vi "analog write with coercion.vi"(6 "write?":bool=TRUE, 8 "error in (no error)":errorcluster, 10 "data":dbl format="%0.2f", 11 "task/channels in":refnum<k21>) -> (0 "error out":errorcluster, 3 "task out":refnum<k21>)   [LabVIEW 2013]
uses:
  <vilib>/DAQmx/write.llb/DAQmx Write (Analog DBL 1Chan 1Samp).vi
  <vilib>/DAQmx/miscellaneous.llb/DAQmx Fill In Error Info.vi
  <resource>/objmgr/daqmx.rc
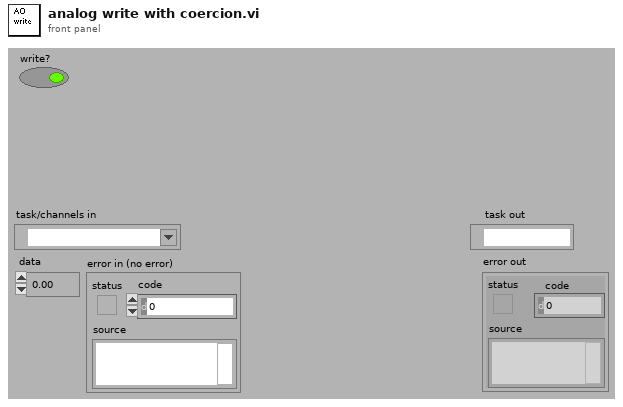
[diagram p1: front panel]
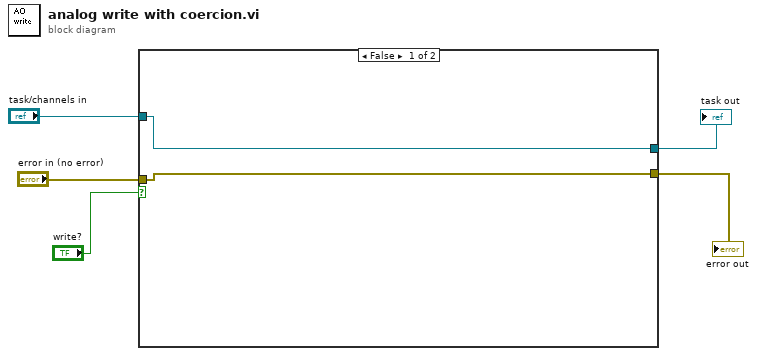
[diagram p0: block diagram]
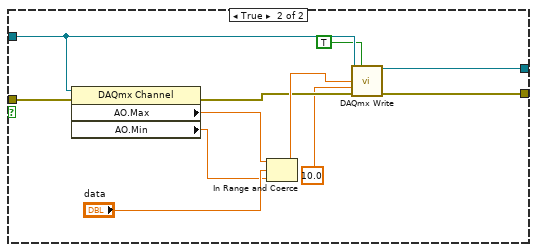
[diagram p2: hidden frame]
diagram:
  n1 = case shown="False" "write?" {
    tunnel: "task/channels in" -> [w7 w18]
    tunnel: [w7 w11] -> w4
    tunnel: [w6 w10] -> w3
    tunnel: "error in (no error)" -> [w6 w8]
    frame False {
    }
    frame True {
      n2 = property class="DAQmx Channel"(reference=w18, error in=w8) -> (error out=w13:errorcluster, "AO.Max"=w15:dbl, "AO.Min"=w16:dbl)  [unwired: 1 out]
      n3 = In Range and Coerce(upper limit=w15, x="data", lower limit=w16) -> (coerced(x)=w14:dbl)  [unwired: 1 out]
      n4 = call-poly <vilib>:"DAQmx Write.vi"("task/channels in"=w18, "auto start"=TRUE, "data"=w14, "timeout"=10.0, "error in"=w13) -> ("task out"=w11:refnum<k21>, "error out"=w10:errorcluster)  [unwired: 8 in, 1 out]
    }
  }
  "task out" <- w4
  "error out" <- w3
